vi "test 11- workerModeCallsWorkerMode.vi"(8 "error in (no error)":errorcluster, 11 "TestCase in":refnum<class "testcase-SyncMessage.lvclass">) -> (0 "error out":errorcluster, 3 "TestCase out":refnum<class "testcase-SyncMessage.lvclass">)   [LabVIEW 2017, in "testcase-SyncMessage.lvclass"]
uses:
  testcase-SyncMessage.lvclass
  <vilib>/addons/_JKI Toolkits/VI Tester/TestCase.llb/TestCase.lvclass
  src/user.lib/_NEVSTOP/Communicable State Machine(CSM)/Communicable State Machine.lvlib
  C:/Program Files (x86)/National Instruments/LabVIEW 2017/vi.lib/addons/_JKI Toolkits/VI Tester/TestCase.llb/TestCase.lvclass
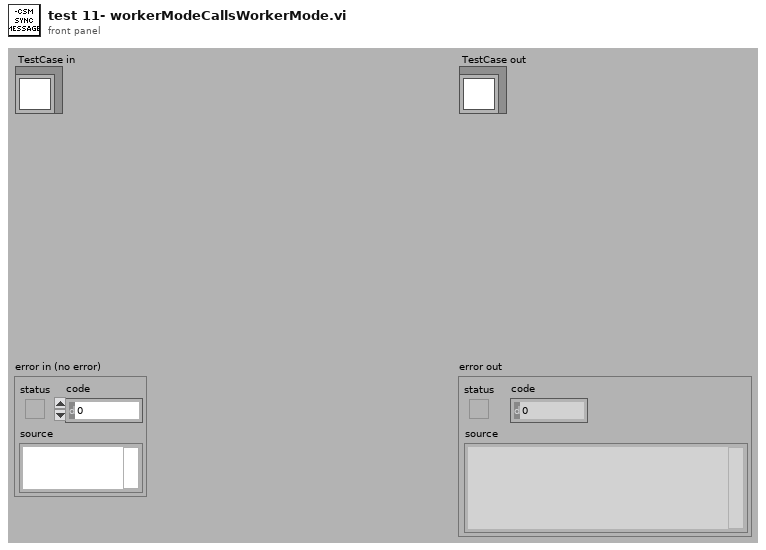
[diagram p1: front panel]
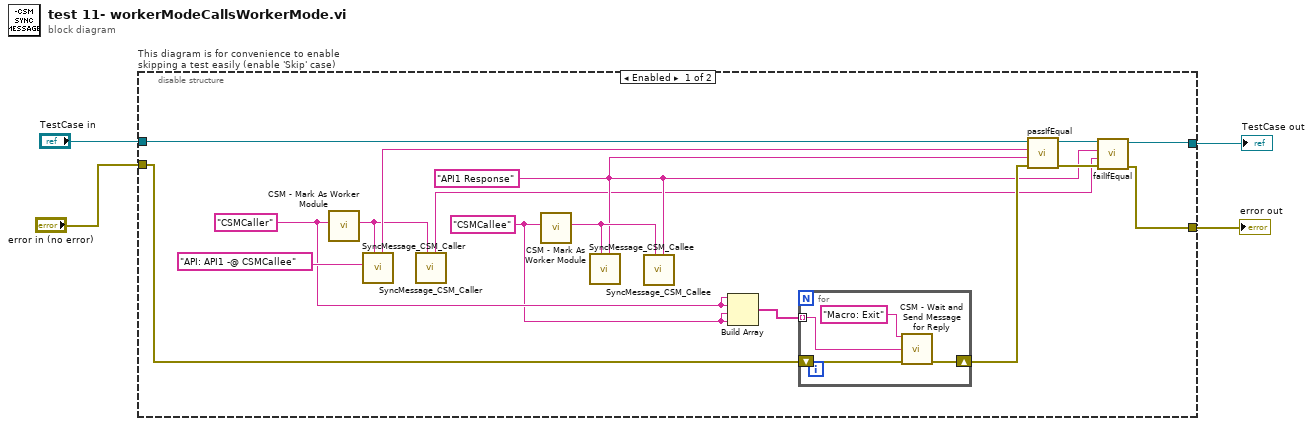
[diagram p0: block diagram]
diagram:
  n1 = disable-structure "This diagram is for convenience to enable skipping a test easily (enable 'Skip' case)" shown="Enabled" {
    disable-tunnel: "TestCase in" -> [w20 w28]
    disable-tunnel: [w9 w26] -> w2
    disable-tunnel: [w7 w27] -> w1
    disable-tunnel: "error in (no error)" -> [w14 w25]
    frame Enabled {
      w11 = "CSMCallee" ("CSMCallee")
      w12 = "CSMCaller" ("CSMCaller")
      w6 = "API1 Response" ("API response in")
      n2 = call "CSM - Mark As Worker Module.vi"("CSM Name"=w12) -> ("CSM Name (Marked As Worker)"=w13:string)  [unwired: 9 in]
      n3 = call "SyncMessage_CSM_Caller.vi"("Name (\"\" to Use UUID)"=w13, "Intermodule Message in"="API: API1 -@ CSMCallee") -> ("API received Response out"=w18:string)  [unwired: 9 in]
      n4 = call "SyncMessage_CSM_Caller.vi"("Name (\"\" to Use UUID)"=w13) -> ("API received Response out"=w5:string)  [unwired: 10 in]
      n5 = call "CSM - Mark As Worker Module.vi"("CSM Name"=w11) -> ("CSM Name (Marked As Worker)"=w15:string)  [unwired: 9 in]
      n6 = call "SyncMessage_CSM_Callee.vi"("API response in"=w6, "Name (\"\" to Use UUID)"=w15) -> ()  [unwired: 10 in]
      n7 = call "SyncMessage_CSM_Callee.vi"("API response in"=w6, "Name (\"\" to Use UUID)"=w15) -> ()  [unwired: 10 in]
      n8 = Build Array(w12, w12, w11, w11) -> (w17:string[])
      n9 = for {
        shift-right: [w22] -> w16
        shift-left: w14 -> [w23]
        tunnel: w17 -> [w21] mode=indexing
        n10 = call "CSM - Wait and Send Message for Reply.vi"("State"="Macro: Exit", "Target Module"=w21, "Error In (No Error)"=w23) -> ("error out"=w22:errorcluster)  [unwired: 10 in, 2 out]
      }
      n11 = call-dynamic "passIfEqual.vi"("error in (no error)"=w16, "y"=w6, "x"=w18, "TestCase in"=w20) -> ("error out"=w8:errorcluster, "TestCase out"=w10:refnum<class "testcase-SyncMessage.lvclass">)  [unwired: 6 in]
      n12 = call-dynamic "failIfEqual.vi"("error in (no error)"=w8, "y"=w5, "x"=w6, "TestCase in"=w10) -> ("error out"=w7:errorcluster, "TestCase out"=w9:refnum<class "testcase-SyncMessage.lvclass">)  [unwired: 6 in]
    }
    frame Disabled {
      # "skip test result while test is under development"
      n13 = call <vilib>:"skip.vi"("error in (no error)"=w25, "TestCase in"=w28) -> ("error out"=w27:errorcluster, "TestCase out"=w26:refnum<class "testcase-SyncMessage.lvclass">)  [unwired: 8 in]
    }
  }
  "error out" <- w1
  "TestCase out" <- w2
